vi "TurnRightXDegrees.vi"() -> ()   [LabVIEW 2019]
uses:
  <vilib>/Rock Robotics/WPI/ThirdParty/Sensors/navX/_TypeDefs/FRIC_navX_DeviceNumbersTypeDef.ctl
  <vilib>/addons/control/pid/pid.llb/PID (DBL).vi
  <vilib>/addons/control/pid/NI_PID_pid.lvlib
panel:
  out "Joystick X":dbl
  in  "Angle (-180 à 180)":dbl
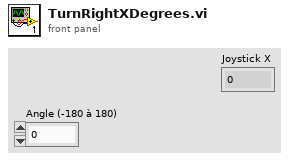
[diagram p1: front panel]
types:
  T1 = typedef "FRIC_navX_DeviceNumbersTypeDef.ctl" = enum16{"Dev0", "Dev1", "Dev2", "Dev3"}
  T2 = cluster{"proportional gain (Kc)":dbl, "integral time (Ti, min)":dbl, "derivative time (Td, min)":dbl}
  T3 = cluster{"Yaw":dbl, "Roll":dbl, "Pitch":dbl, "Heading":dbl, "Fused Heading":dbl}
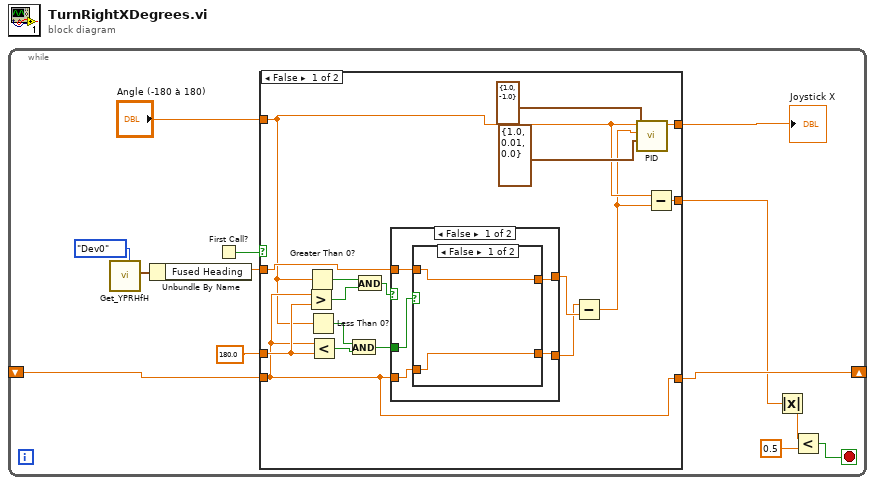
[diagram p0: block diagram]
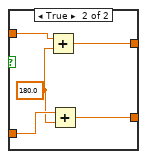
[diagram p2: hidden frame]
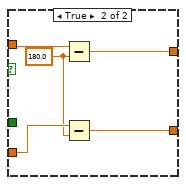
[diagram p3: hidden frame]
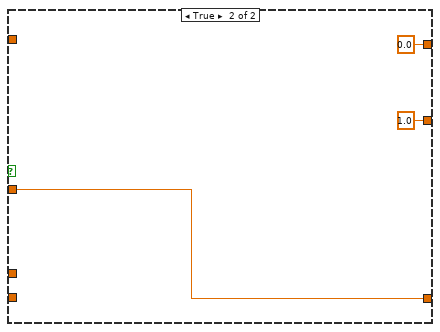
[diagram p4: hidden frame]
diagram:
  n1 = while {
    shift-right: [w9] -> _
    shift-left: _ -> [w8]
    stop <- w4 stop-if-true
    n2 = call <vilib>:"Get_YPRHfH.vi"("Device Number"=FRIC_navX_DeviceNumbersTypeDef."Dev0") -> ("YRPHfH"=w12:T3)  [unwired: 10 in]
    n3 = Unbundle By Name(w12) -> ("Fused Heading"=w10:dbl)
    n4 = First Call?() -> (First Call?: T/F=w11:bool)
    n5 = case shown="False" w11 {
      tunnel: w10 -> [w21 w50]
      tunnel: [w18 w50] -> w9
      tunnel: w8 -> [w18 _]
      tunnel: "Angle (-180 à 180)" -> [w16 _]
      tunnel: 180.0 ("x") -> [w24 _]
      tunnel: [w17 0.0 ("output")] -> w5
      tunnel: [w14 1.0] -> w3
      frame False {
        n6 = Greater?(x=w18, y=w24) -> (0:w25:bool)
        n7 = Greater Than 0?(x=w16) -> (x > 0?=w26:bool)
        n8 = Less Than 0?(x=w16) -> (x < 0?=w27:bool)
        n9 = Less?(x=w18, y=w24) -> (x < y?=w28:bool)
        n10 = And(x=w27, y=w28) -> (x .and. y?=w22:bool)
        n11 = And(x=w26, y=w25) -> (x .and. y?=w23:bool)
        n12 = case shown="False" w23 {
          tunnel: w22 -> [w35 _]
          tunnel: w21 -> [w33 w46]
          tunnel: w18 -> [w34 w47]
          tunnel: [w31 w44] -> w19
          tunnel: [w32 w43] -> w20
          frame False {
            n13 = case shown="False" w35 {
              tunnel: w34 -> [w37 w42]
              tunnel: w33 -> [w36 w41]
              tunnel: [w36 w39] -> w32
              tunnel: [w37 w38] -> w31
              frame False {
              }
              frame True {
                w40 = 180.0 ("y")
                n14 = Add(x=w41, y=w40) -> (x+y=w39:dbl)
                n15 = Add(x=w42, y=w40) -> (x+y=w38:dbl)
              }
            }
          }
          frame True {
            w45 = 180.0 ("y")
            n16 = Subtract(x=w46, y=w45) -> (x-y=w43:dbl)
            n17 = Subtract(x=w47, y=w45) -> (x-y=w44:dbl)
          }
        }
        n18 = Subtract(x=w19, y=w20) -> (x-y=w15:dbl)
        n19 = call-poly <vilib>:"PID.vi"("output range"=cluster{"output high":dbl, "output low":dbl} {"output high"=1.0, "output low"=-1.0}, "PID gains"=T2 {"proportional gain (Kc)"=1.0, "integral time (Ti, min)"=0.01, "derivative time (Td, min)"=0.0}, "process variable"=w15, "setpoint"=w16) -> ("output"=w17:dbl)  [unwired: 6 in, 1 out]
        n20 = Subtract(x=w16, y=w15) -> (x-y=w14:dbl)
      }
      frame True {
      }
    }
    "Joystick X" <- w5
    n21 = Absolute Value(x=w3) -> (abs(x)=w1:dbl)
    n22 = Less?(x=w1, y=0.5) -> (x < y?=w4:bool)
  }
